vi "Run.vi"(8 "error in (no error)":errorcluster, 11 "Model Index":i32) -> (0 "error out":errorcluster, 3 "Return":i32)   [LabVIEW 2015]
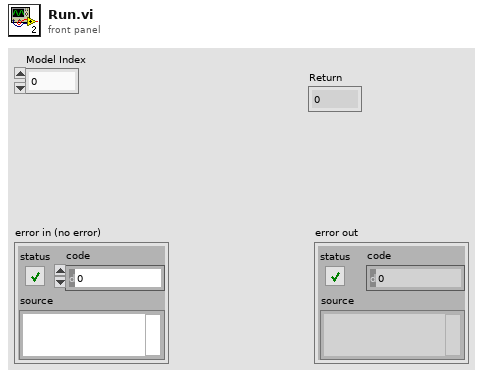
[diagram p1: front panel]
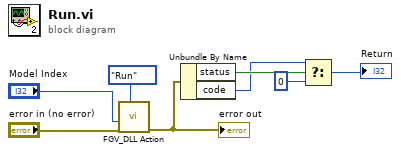
[diagram p0: block diagram]
diagram:
  n1 = call "FGV_DLL Action.vi"("State"=enum16{"Initial", "Run", "Close"}."Run", "Error In"="error in (no error)", "Model Index"="Model Index") -> ("Error Out"=w1:errorcluster)  [unwired: 8 in]
  "error out" <- w1
  n2 = Unbundle By Name(w1) -> ("status"=w5:bool, "code"=w4:i32)
  n3 = Select(t=w4, s=w5, f=0) -> (s? t:f=→"Return":i32)
